vi "getPathOfTestLvLib.vi"() -> (3 "testLvLibPath":path)   [LabVIEW 2018]
doc: "Get the test file path of LabVIEW library."
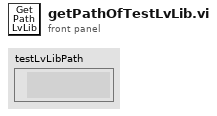
[diagram p1: front panel]
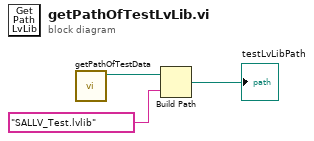
[diagram p0: block diagram]
diagram:
  n1 = call "getPathOfTestData.vi"() -> ("testDataPath"=w3:path)  [unwired: 11 in]
  n2 = Build Path(base path=w3, name or relative path="SALLV_Test.lvlib") -> (appended path=→"testLvLibPath":path)
